vi "Nattify - Get Window Margins.vi"(11 "error in":errorcluster) -> (4 "window margins":T1, 15 "error out":errorcluster)   [LabVIEW 2020]
uses:
  Nattify - Window Margins.ctl
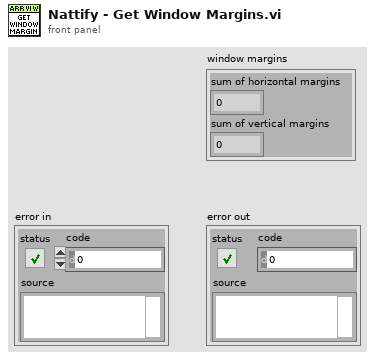
[diagram p1: front panel]
types:
  T1 = typedef "Nattify - Window Margins.ctl" = cluster{"sum of horizontal margins":i16, "sum of vertical margins":i16}
  T2 = typedef "LVRectTypeDef.ctl" = cluster{"Left":i16, "Top":i16, "Right":i16, "Bottom":i16}
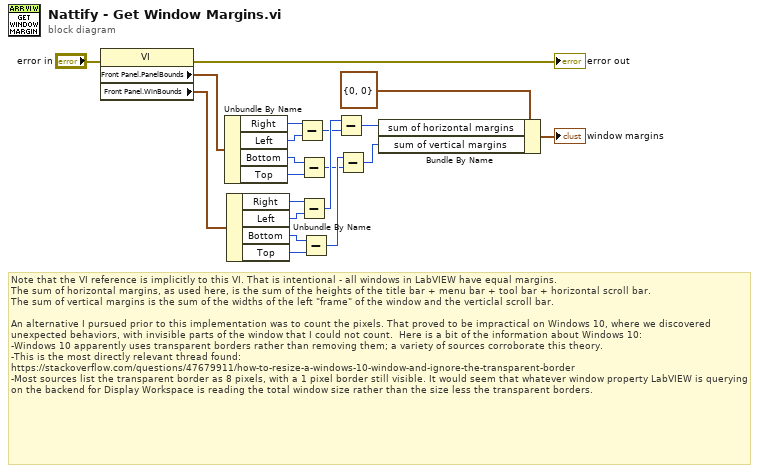
[diagram p0: block diagram]
diagram:
  # "Note that the VI reference is implicitly to this VI. That is intentional - all windows in LabVIEW have equal margins.\nThe sum of horizontal margins, as used here, is the sum of the heights of the title bar + menu bar + tool bar + horizontal scroll bar.\nThe sum of vertical margins is the sum of the widths of the left \"frame\" of the window and the verticlal scroll bar.\n\nAn alternative I pursued prior to this implementation was to count the pixels. That proved to be impractical on Windows 10, where we discovered unexpected behaviors, with invisible parts of the window that I could not count.  Here is a bit of the information about Windows 10:\n-Windows 10 apparently uses transparent borders rather than removing them; a variety of sources corroborate this theory.\n-This is the most directly relevant thread found:\nhttps://stackoverflow.com/questions/47679911/how-to-resize-a-windows-10-window-and-ignore-the-transparent-border \n-Most sources list the transparent border as 8 pixels, with a 1 pixel border still visible. It would seem that whatever window property LabVIEW is querying on the backend for Display Workspace is reading the total window size rather than the size less the transparent borders."
  n1 = property on="Property Node" class="VI"(error in="error in") -> (error out=→"error out":errorcluster, "Front Panel.PanelBounds"=w5:T2, "Front Panel.WinBounds"=w12:T2)  [unwired: 1 in, 1 out]
  n2 = Unbundle By Name(w5) -> ("Right"=w20:i16, "Left"=w19:i16, "Bottom"=w18:i16, "Top"=w17:i16)
  n3 = Unbundle By Name(w12) -> ("Right"=w13:i16, "Left"=w14:i16, "Bottom"=w15:i16, "Top"=w16:i16)
  n4 = Subtract(x=w20, y=w19) -> (x-y=w10:i16)
  n5 = Subtract(x=w18, y=w17) -> (x-y=w8:i16)
  n6 = Subtract(x=w13, y=w14) -> (x-y=w11:i16)
  n7 = Subtract(x=w15, y=w16) -> (x-y=w9:i16)
  n8 = Subtract(x=w11, y=w10) -> (x-y=w3:i16)
  n9 = Subtract(x=w9, y=w8) -> (x-y=w2:i16)
  n10 = Bundle By Name(cluster=T1 {"sum of horizontal margins"=0, "sum of vertical margins"=0} ("window margins"), "sum of horizontal margins"=w3, "sum of vertical margins"=w2) -> (→"window margins":T1)
